vi "Begin.vi"(8 "error in":errorcluster) -> (0 "error out":errorcluster)   [LabVIEW 2018]
doc: "Called before other user functions, this VI is expected to open initial I/O refnums, load in file data, and do all program initialization. Notice that the <B>error out</B> terminal is simply used for data flow. Wiring it to other structures or subVIs ensures that this VI runs first."
uses:
  <vilib>/Rock Robotics/WPI/DriverStation/WPI_DriverStationRobotMode2.ctl
  <vilib>/Rock Robotics/WPI/Joystick/WPI_JoystickDeviceEnum.ctl
  <vilib>/Rock Robotics/WPI/Solenoid/WPI_SolenoidChannel.ctl
  <vilib>/Rock Robotics/SystemInterfaces/DIO/FPGA_DIOChannel.ctl
  <vilib>/Rock Robotics/SystemInterfaces/DIO/FPGA_DIOPWMChannel.ctl
  Robot Global Data.vi
  <vilib>/Rock Robotics/WPI/Solenoid/WPI_SolenoidOpenSingle.vi
  <vilib>/Rock Robotics/WPI/Switch/WPI_SwitchOpenLimit.vi
  <vilib>/Rock Robotics/WPI/Utilities/WPI_GetSetVariantRefNum.vi
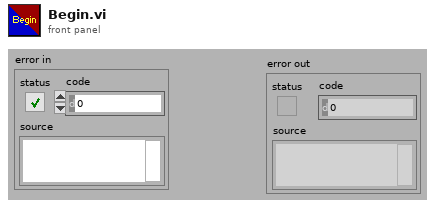
[diagram p1: front panel]
types:
  T1 = typedef "FPGA_DIOPWMChannel.ctl" = enum8{"PWM 0", "PWM 1", "PWM 2", "PWM 3", "PWM 4", "PWM 5", "PWM 6", "PWM 7", "PWM 8", "PWM 9", "PWM MXP 0", "PWM MXP 1", "PWM MXP 2", "PWM MXP 3", "PWM MXP 4", "PWM MXP 5", "PWM MXP 6", "PWM MXP 7", "PWM MXP 8", "PWM MXP 9", "Invalid"}
  T2 = typedef "FPGA_DIOChannel.ctl" = enum8{"DIO 0", "DIO 1", "DIO 2", "DIO 3", "DIO 4", "DIO 5", "DIO 6", "DIO 7", "DIO 8", "DIO 9", "DIO MXP 0", "DIO MXP 1", "DIO MXP 2", "DIO MXP 3", "DIO MXP 4", "DIO MXP 5", "DIO MXP 6", "DIO MXP 7", "DIO MXP 8", "DIO MXP 9", "DIO MXP 10", "DIO MXP 11", "DIO MXP 12", "DIO MXP 13", "DIO MXP 14", "DIO MXP 15", "SPI Port CS1", "SPI Port CS2", "SPI Port CS3", "SPI Port MISO", "SPI Port MOSI", "Invalid"}
  T3 = typedef "WPI_SolenoidChannel.ctl" = enum8{"Solenoid 0", "Solenoid 1", "Solenoid 2", "Solenoid 3", "Solenoid 4", "Solenoid 5", "Solenoid 6", "Solenoid 7", "Invalid"}
  T4 = typedef "WPI_JoystickDeviceEnum.ctl" = enum16{"USB 0", "USB 1", "USB 2", "USB 3", "USB 4", "USB 5"}
  T5 = typedef "WPI_DriverStationRobotMode2.ctl" = enum16{"Autonomous Disabled", "Autonomous Enabled", "Teleop Disabled", "Teleop Enabled", "Disconnected", "Finish", "Test Disabled", "Test Enabled", "Emergency Stopped"}
  T6 = typedef "WPI_MotorControlDeviceRef.ctl" = cluster{"DeviceStatus":errorcluster, "Type":T7, "PWM":cluster{"PWM Channel":T1, "DeadBand":T8}, "CAN":cluster{"Device Number":u8, "SetOutput VI Ref":variant, "GetOutput VI Ref":variant, "Enable VI Ref":variant, "Disable VI Ref":variant, "Data":variant}, "Invert":bool, "DIO PWM":cluster{"PWM \"Enable\" Channel":T1, "DIOChannel":T2, "PWM Rate":dbl}}
  T7 = typedef "WPI_MotorControlType.ctl" = enum16{"PWM", "CAN", "DIO PWM"}
  T8 = typedef "WPI_PWMDeadband.ctl" = cluster{"Name":string, "maxPositivePwm":i32, "minPositivePwm":i32, "centerPwm":i32, "maxNegativePwm":i32, "minNegativePwm":i32, "angularRange":u16}
  T9 = typedef "WPI_JoystickDevRef.ctl" = cluster{"Device":T4}
  T10 = typedef "WPI_SwitchDevRef.ctl" = cluster{"DevStatus":errorcluster, "DIO Channel":T2, "CntIndex":T11, "Normally Closed":bool}
  T11 = typedef "FPGA_CounterCtrSystemIndex.ctl" = enum8{"Ctr 0", "Ctr 1", "Ctr 2", "Ctr 3", "Ctr 4", "Ctr 5", "Ctr 6", "Ctr 7", "Invalid"}
  T12 = typedef "WPI_CompressorDevRef.ctl" = cluster{"DevStatus":errorcluster, "Pneumatics Control Module":u8}
  T13 = typedef "WPI_SolenoidDevRef.ctl" = cluster{"DevStatus":errorcluster, "Pneumatics Control Module":u8, "Forward Solenoid Channel":T3, "Reverse Solenoid Channel":T3}
  T14 = typedef "WPI_PWMDeviceRef.ctl" = cluster{"DeviceStatus":errorcluster, "PWM Channel":T1}
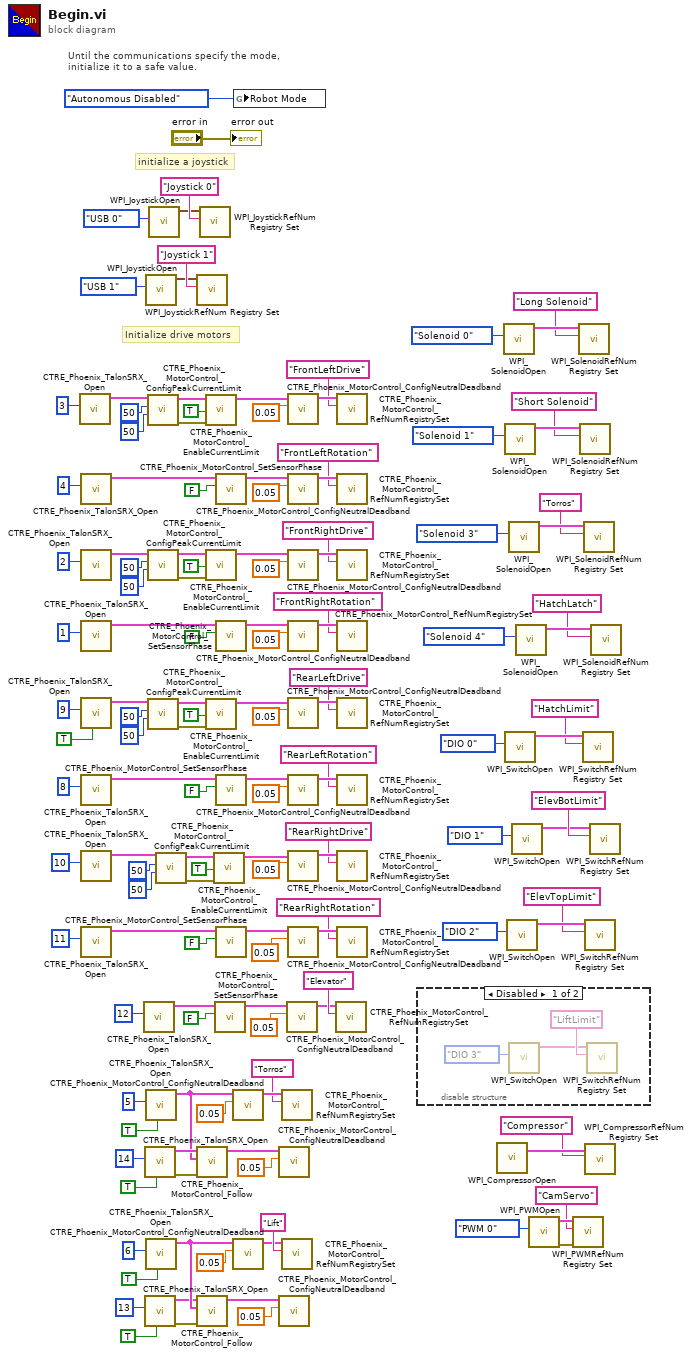
[diagram p0: block diagram]
diagram:
  # "Initialize drive motors"
  # "initialize a joystick"
  # "Until the communications specify the mode,\ninitialize it to a safe value."
  n1 = call <vilib>:"CTRE_Phoenix_TalonSRX_Open.vi"("Device Number"=u8 3) -> ("CAN Talon SRX Ref"=w19:T6)  [unwired: 9 in, 1 out]
  n2 = call <vilib>:"CTRE_Phoenix_TalonSRX_Open.vi"("Device Number"=u8 4) -> ("CAN Talon SRX Ref"=w129:T6)  [unwired: 9 in, 1 out]
  n3 = call <vilib>:"CTRE_Phoenix_TalonSRX_Open.vi"("Device Number"=u8 2) -> ("CAN Talon SRX Ref"=w25:T6)  [unwired: 9 in, 1 out]
  n4 = call <vilib>:"CTRE_Phoenix_TalonSRX_Open.vi"("Device Number"=u8 1) -> ("CAN Talon SRX Ref"=w118:T6)  [unwired: 9 in, 1 out]
  n5 = call <vilib>:"CTRE_Phoenix_TalonSRX_Open.vi"("Invert"=TRUE, "Device Number"=u8 9) -> ("CAN Talon SRX Ref"=w23:T6)  [unwired: 8 in, 1 out]
  n6 = call <vilib>:"CTRE_Phoenix_TalonSRX_Open.vi"("Device Number"=u8 8) -> ("CAN Talon SRX Ref"=w108:T6)  [unwired: 9 in, 1 out]
  n7 = call <vilib>:"CTRE_Phoenix_TalonSRX_Open.vi"("Device Number"=u8 10) -> ("CAN Talon SRX Ref"=w21:T6)  [unwired: 9 in, 1 out]
  n8 = call <vilib>:"CTRE_Phoenix_TalonSRX_Open.vi"("Device Number"=u8 11) -> ("CAN Talon SRX Ref"=w91:T6)  [unwired: 9 in, 1 out]
  n9 = call <vilib>:"CTRE_Phoenix_TalonSRX_Open.vi"("Device Number"=u8 12) -> ("CAN Talon SRX Ref"=w73:T6)  [unwired: 9 in, 1 out]
  n10 = call <vilib>:"CTRE_Phoenix_TalonSRX_Open.vi"("Invert"=TRUE, "Device Number"=u8 14) -> ("error out"=w56:errorcluster, "CAN Talon SRX Ref"=w55:T6)  [unwired: 8 in]
  n11 = call <vilib>:"CTRE_Phoenix_TalonSRX_Open.vi"("Invert"=TRUE, "Device Number"=u8 13) -> ("error out"=w13:errorcluster, "CAN Talon SRX Ref"=w14:T6)  [unwired: 8 in]
  n12 = call <vilib>:"WPI_JoystickOpen.vi"("JoystickDevice"=WPI_JoystickDeviceEnum."USB 1") -> ("JoystickDevRef"=w88:T9)  [unwired: 10 in]
  n13 = call <vilib>:"CTRE_Phoenix_TalonSRX_Open.vi"("Invert"=TRUE, "Device Number"=u8 5) -> ("CAN Talon SRX Ref"=w54:T6)  [unwired: 8 in, 1 out]
  n14 = call <vilib>:"CTRE_Phoenix_TalonSRX_Open.vi"("Invert"=TRUE, "Device Number"=u8 6) -> ("CAN Talon SRX Ref"=w15:T6)  [unwired: 8 in, 1 out]
  n15 = call <vilib>:"CTRE_Phoenix_MotorControl_ConfigPeakCurrentLimit.vi"("Peak Current Maximum Duration (ms)"=50, "Peak Current (Amps)"=50, "PhoenixMotorControlDevRef"=w19) -> ("error out"=w26:errorcluster, "PhoenixMotorControlDevRef"=w27:T6)  [unwired: 7 in]
  n16 = call <vilib>:"CTRE_Phoenix_MotorControl_ConfigPeakCurrentLimit.vi"("Peak Current Maximum Duration (ms)"=50, "Peak Current (Amps)"=50, "PhoenixMotorControlDevRef"=w25) -> ("error out"=w35:errorcluster, "PhoenixMotorControlDevRef"=w34:T6)  [unwired: 7 in]
  n17 = call <vilib>:"CTRE_Phoenix_MotorControl_ConfigPeakCurrentLimit.vi"("Peak Current Maximum Duration (ms)"=50, "Peak Current (Amps)"=50, "PhoenixMotorControlDevRef"=w23) -> ("error out"=w36:errorcluster, "PhoenixMotorControlDevRef"=w37:T6)  [unwired: 7 in]
  n18 = call <vilib>:"WPI_JoystickOpen.vi"("JoystickDevice"=WPI_JoystickDeviceEnum."USB 0") -> ("JoystickDevRef"=w137:T9)  [unwired: 10 in]
  n19 = call <vilib>:"CTRE_Phoenix_MotorControl_ConfigPeakCurrentLimit.vi"("Peak Current Maximum Duration (ms)"=50, "Peak Current (Amps)"=50, "PhoenixMotorControlDevRef"=w21) -> ("error out"=w45:errorcluster, "PhoenixMotorControlDevRef"=w44:T6)  [unwired: 7 in]
  n20 = call <vilib>:"WPI_JoystickRefNum Registry Set.vi"("refnum name"="Joystick 1", "JoystickDevRef"=w88) -> ()  [unwired: 8 in, 2 out]
  n21 = call <vilib>:"CTRE_Phoenix_MotorControl_Follow.vi"("error in (no error)"=w56, "Master Controller to Follow"=w54, "PhoenixMotorControlDevRef"=w55) -> ("PhoenixMotorControlDevRef"=w53:T6)  [unwired: 7 in, 1 out]
  n22 = call <vilib>:"CTRE_Phoenix_MotorControl_Follow.vi"("error in (no error)"=w13, "Master Controller to Follow"=w15, "PhoenixMotorControlDevRef"=w14) -> ("PhoenixMotorControlDevRef"=w16:T6)  [unwired: 7 in, 1 out]
  n23 = call <vilib>:"WPI_JoystickRefNum Registry Set.vi"("refnum name"="Joystick 0", "JoystickDevRef"=w137) -> ()  [unwired: 8 in, 2 out]
  n24 = call <vilib>:"CTRE_Phoenix_MotorControl_EnableCurrentLimit.vi"("error in (no error)"=w26, "Enable Current Limit?"=TRUE, "PhoenixMotorControlDevRef"=w27) -> ("PhoenixMotorControlDevRef"=w18:T6)  [unwired: 7 in, 1 out]
  n25 = call <vilib>:"CTRE_Phoenix_MotorControl_EnableCurrentLimit.vi"("error in (no error)"=w35, "Enable Current Limit?"=TRUE, "PhoenixMotorControlDevRef"=w34) -> ("PhoenixMotorControlDevRef"=w24:T6)  [unwired: 7 in, 1 out]
  n26 = call <vilib>:"CTRE_Phoenix_MotorControl_EnableCurrentLimit.vi"("error in (no error)"=w36, "Enable Current Limit?"=TRUE, "PhoenixMotorControlDevRef"=w37) -> ("PhoenixMotorControlDevRef"=w22:T6)  [unwired: 7 in, 1 out]
  n27 = call <vilib>:"CTRE_Phoenix_MotorControl_EnableCurrentLimit.vi"("error in (no error)"=w45, "Enable Current Limit?"=TRUE, "PhoenixMotorControlDevRef"=w44) -> ("PhoenixMotorControlDevRef"=w20:T6)  [unwired: 7 in, 1 out]
  n28 = call <vilib>:"CTRE_Phoenix_MotorControl_SetSensorPhase.vi"("PhaseSensor"=FALSE, "PhoenixMotorControlDevRef"=w73) -> ("PhoenixMotorControlDevRef"=w70:T6)  [unwired: 8 in, 1 out]
  n29 = call <vilib>:"CTRE_Phoenix_MotorControl_SetSensorPhase.vi"("PhaseSensor"=FALSE, "PhoenixMotorControlDevRef"=w129) -> ("PhoenixMotorControlDevRef"=w131:T6)  [unwired: 8 in, 1 out]
  n30 = call <vilib>:"CTRE_Phoenix_MotorControl_SetSensorPhase.vi"("PhaseSensor"=FALSE, "PhoenixMotorControlDevRef"=w118) -> ("PhoenixMotorControlDevRef"=w117:T6)  [unwired: 8 in, 1 out]
  n31 = call <vilib>:"CTRE_Phoenix_MotorControl_SetSensorPhase.vi"("PhaseSensor"=FALSE, "PhoenixMotorControlDevRef"=w108) -> ("PhoenixMotorControlDevRef"=w109:T6)  [unwired: 8 in, 1 out]
  n32 = call <vilib>:"CTRE_Phoenix_MotorControl_SetSensorPhase.vi"("PhaseSensor"=FALSE, "PhoenixMotorControlDevRef"=w91) -> ("PhoenixMotorControlDevRef"=w100:T6)  [unwired: 8 in, 1 out]
  n33 = call <vilib>:"CTRE_Phoenix_MotorControl_ConfigNeutralDeadband.vi"("Percent Deadband"=0.05, "PhoenixMotorControlDevRef"=w54) -> ("PhoenixMotorControlDevRef"=w61:T6)  [unwired: 8 in, 1 out]
  n34 = call <vilib>:"CTRE_Phoenix_MotorControl_ConfigNeutralDeadband.vi"("Percent Deadband"=0.05, "PhoenixMotorControlDevRef"=w15) -> ("PhoenixMotorControlDevRef"=w8:T6)  [unwired: 8 in, 1 out]
  n35 = global write "Robot Global Data.vi" "Robot Mode"(WPI_DriverStationRobotMode2."Autonomous Disabled" ("Robot Mode")) -> ()
  n36 = call <vilib>:"CTRE_Phoenix_MotorControl_ConfigNeutralDeadband.vi"("Percent Deadband"=0.05, "PhoenixMotorControlDevRef"=w53) -> ()  [unwired: 8 in, 2 out]
  n37 = call <vilib>:"CTRE_Phoenix_MotorControl_ConfigNeutralDeadband.vi"("Percent Deadband"=0.05, "PhoenixMotorControlDevRef"=w16) -> ()  [unwired: 8 in, 2 out]
  n38 = call <vilib>:"CTRE_Phoenix_MotorControl_RefNumRegistrySet.vi"("refnum name"="Torros", "PhoenixMotorControlDevRef"=w61) -> ()  [unwired: 8 in, 2 out]
  n39 = call <vilib>:"CTRE_Phoenix_MotorControl_RefNumRegistrySet.vi"("refnum name"="Lift", "PhoenixMotorControlDevRef"=w8) -> ()  [unwired: 8 in, 2 out]
  n40 = call <vilib>:"CTRE_Phoenix_MotorControl_ConfigNeutralDeadband.vi"("Percent Deadband"=0.05, "PhoenixMotorControlDevRef"=w70) -> ("PhoenixMotorControlDevRef"=w71:T6)  [unwired: 8 in, 1 out]
  n41 = call <vilib>:"CTRE_Phoenix_MotorControl_ConfigNeutralDeadband.vi"("Percent Deadband"=0.05, "PhoenixMotorControlDevRef"=w18) -> ("PhoenixMotorControlDevRef"=w130:T6)  [unwired: 8 in, 1 out]
  n42 = call <vilib>:"CTRE_Phoenix_MotorControl_ConfigNeutralDeadband.vi"("Percent Deadband"=0.05, "PhoenixMotorControlDevRef"=w131) -> ("PhoenixMotorControlDevRef"=w128:T6)  [unwired: 8 in, 1 out]
  n43 = call <vilib>:"CTRE_Phoenix_MotorControl_ConfigNeutralDeadband.vi"("Percent Deadband"=0.05, "PhoenixMotorControlDevRef"=w24) -> ("PhoenixMotorControlDevRef"=w122:T6)  [unwired: 8 in, 1 out]
  n44 = call <vilib>:"CTRE_Phoenix_MotorControl_ConfigNeutralDeadband.vi"("Percent Deadband"=0.05, "PhoenixMotorControlDevRef"=w117) -> ("PhoenixMotorControlDevRef"=w119:T6)  [unwired: 8 in, 1 out]
  n45 = call <vilib>:"CTRE_Phoenix_MotorControl_ConfigNeutralDeadband.vi"("Percent Deadband"=0.05, "PhoenixMotorControlDevRef"=w22) -> ("PhoenixMotorControlDevRef"=w113:T6)  [unwired: 8 in, 1 out]
  n46 = call <vilib>:"CTRE_Phoenix_MotorControl_ConfigNeutralDeadband.vi"("Percent Deadband"=0.05, "PhoenixMotorControlDevRef"=w109) -> ("PhoenixMotorControlDevRef"=w107:T6)  [unwired: 8 in, 1 out]
  n47 = call <vilib>:"CTRE_Phoenix_MotorControl_ConfigNeutralDeadband.vi"("Percent Deadband"=0.05, "PhoenixMotorControlDevRef"=w20) -> ("PhoenixMotorControlDevRef"=w104:T6)  [unwired: 8 in, 1 out]
  n48 = call <vilib>:"CTRE_Phoenix_MotorControl_ConfigNeutralDeadband.vi"("Percent Deadband"=0.05, "PhoenixMotorControlDevRef"=w100) -> ("PhoenixMotorControlDevRef"=w99:T6)  [unwired: 8 in, 1 out]
  n49 = call <vilib>:"CTRE_Phoenix_MotorControl_RefNumRegistrySet.vi"("refnum name"="Elevator", "PhoenixMotorControlDevRef"=w71) -> ()  [unwired: 8 in, 2 out]
  n50 = call <vilib>:"CTRE_Phoenix_MotorControl_RefNumRegistrySet.vi"("refnum name"="FrontLeftDrive", "PhoenixMotorControlDevRef"=w130) -> ()  [unwired: 8 in, 2 out]
  n51 = call <vilib>:"CTRE_Phoenix_MotorControl_RefNumRegistrySet.vi"("refnum name"="FrontLeftRotation", "PhoenixMotorControlDevRef"=w128) -> ()  [unwired: 8 in, 2 out]
  n52 = call <vilib>:"CTRE_Phoenix_MotorControl_RefNumRegistrySet.vi"("refnum name"="FrontRightDrive", "PhoenixMotorControlDevRef"=w122) -> ()  [unwired: 8 in, 2 out]
  n53 = call <vilib>:"CTRE_Phoenix_MotorControl_RefNumRegistrySet.vi"("refnum name"="FrontRightRotation", "PhoenixMotorControlDevRef"=w119) -> ()  [unwired: 8 in, 2 out]
  n54 = call <vilib>:"CTRE_Phoenix_MotorControl_RefNumRegistrySet.vi"("refnum name"="RearLeftDrive", "PhoenixMotorControlDevRef"=w113) -> ()  [unwired: 8 in, 2 out]
  n55 = call <vilib>:"CTRE_Phoenix_MotorControl_RefNumRegistrySet.vi"("refnum name"="RearLeftRotation", "PhoenixMotorControlDevRef"=w107) -> ()  [unwired: 8 in, 2 out]
  n56 = call <vilib>:"CTRE_Phoenix_MotorControl_RefNumRegistrySet.vi"("refnum name"="RearRightDrive", "PhoenixMotorControlDevRef"=w104) -> ()  [unwired: 8 in, 2 out]
  n57 = call <vilib>:"CTRE_Phoenix_MotorControl_RefNumRegistrySet.vi"("refnum name"="RearRightRotation", "PhoenixMotorControlDevRef"=w99) -> ()  [unwired: 8 in, 2 out]
  n58 = disable-structure shown="Disabled" {
    frame Disabled {
      n59 = call-poly <vilib>:"WPI_SwitchOpen.vi"("DIO Channel"=FPGA_DIOChannel."DIO 3") -> ("SwitchDevRef"=w140:T10)  [unwired: 9 in, 1 out]
      n60 = call <vilib>:"WPI_SwitchRefNum Registry Set.vi"("refnum name"="LiftLimit", "SwitchDevRef"=w140) -> ()  [unwired: 8 in, 2 out]
    }
    frame Enabled {
    }
  }
  n61 = call <vilib>:"WPI_CompressorOpen.vi"() -> ("CompressorDevRef"=w64:T12)  [unwired: 14 in, 1 out]
  n62 = call-poly <vilib>:"WPI_SolenoidOpen.vi"("Solenoid Channel"=WPI_SolenoidChannel."Solenoid 0") -> ("SolenoidDevRef"=w84:T13)  [unwired: 9 in, 1 out]
  n63 = call-poly <vilib>:"WPI_SolenoidOpen.vi"("Solenoid Channel"=WPI_SolenoidChannel."Solenoid 1") -> ("SolenoidDevRef"=w85:T13)  [unwired: 9 in, 1 out]
  n64 = call-poly <vilib>:"WPI_SwitchOpen.vi"("DIO Channel"=FPGA_DIOChannel."DIO 0") -> ("SwitchDevRef"=w67:T10)  [unwired: 9 in, 1 out]
  n65 = call-poly <vilib>:"WPI_SwitchOpen.vi"("DIO Channel"=FPGA_DIOChannel."DIO 2") -> ("SwitchDevRef"=w49:T10)  [unwired: 9 in, 1 out]
  n66 = call-poly <vilib>:"WPI_SolenoidOpen.vi"("Solenoid Channel"=WPI_SolenoidChannel."Solenoid 3") -> ("SolenoidDevRef"=w78:T13)  [unwired: 9 in, 1 out]
  n67 = call-poly <vilib>:"WPI_SwitchOpen.vi"("DIO Channel"=FPGA_DIOChannel."DIO 1") -> ("SwitchDevRef"=w50:T10)  [unwired: 9 in, 1 out]
  n68 = call-poly <vilib>:"WPI_SolenoidOpen.vi"("Solenoid Channel"=WPI_SolenoidChannel."Solenoid 4") -> ("SolenoidDevRef"=w80:T13)  [unwired: 9 in, 1 out]
  n69 = call <vilib>:"WPI_PWMOpen.vi"("PWM Channel"=FPGA_DIOPWMChannel."PWM 0") -> ("error out"=w6:errorcluster, "PWMDeviceRef"=w5:T14)  [unwired: 9 in]
  n70 = call <vilib>:"WPI_PWMRefNum Registry Set.vi"("error in (no error)"=w6, "refnum name"="CamServo", "PWMDeviceRef"=w5) -> ()  [unwired: 7 in, 2 out]
  n71 = call <vilib>:"WPI_SolenoidRefNum Registry Set.vi"("refnum name"="Long Solenoid", "SolenoidDevRef"=w84) -> ()  [unwired: 8 in, 2 out]
  n72 = call <vilib>:"WPI_SolenoidRefNum Registry Set.vi"("refnum name"="Short Solenoid", "SolenoidDevRef"=w85) -> ()  [unwired: 8 in, 2 out]
  n73 = call <vilib>:"WPI_SwitchRefNum Registry Set.vi"("refnum name"="HatchLimit", "SwitchDevRef"=w67) -> ()  [unwired: 8 in, 2 out]
  n74 = call <vilib>:"WPI_SolenoidRefNum Registry Set.vi"("refnum name"="Torros", "SolenoidDevRef"=w78) -> ()  [unwired: 8 in, 2 out]
  n75 = call <vilib>:"WPI_SwitchRefNum Registry Set.vi"("refnum name"="ElevTopLimit", "SwitchDevRef"=w49) -> ()  [unwired: 8 in, 2 out]
  n76 = call <vilib>:"WPI_CompressorRefNum Registry Set.vi"("refnum name"="Compressor", "CompressorDevRef"=w64) -> ()  [unwired: 8 in, 2 out]
  n77 = call <vilib>:"WPI_SwitchRefNum Registry Set.vi"("refnum name"="ElevBotLimit", "SwitchDevRef"=w50) -> ()  [unwired: 8 in, 2 out]
  n78 = call <vilib>:"WPI_SolenoidRefNum Registry Set.vi"("refnum name"="HatchLatch", "SolenoidDevRef"=w80) -> ()  [unwired: 8 in, 2 out]
  "error out" <- "error in"
